vi "ArrangeNodes.vi"() -> ()   [LabVIEW 2016]
uses:
  <resource>/Framework/Providers/Open_GDS/UML/ArrangeNodes/private/localVar.ctl
panel:
  out "Picture":picture
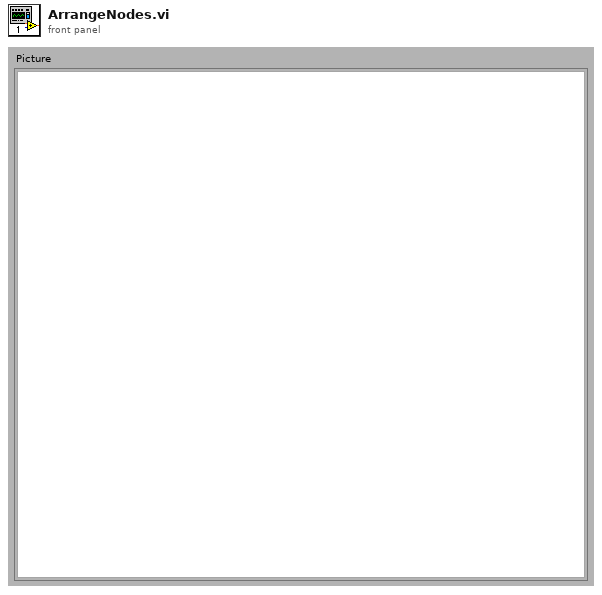
[diagram p1: front panel]
types:
  T1 = typedef "localVar.ctl" = cluster{"nodes":cluster{"x":dbl, "y":dbl, "w":dbl, "h":dbl, "dx":dbl, "dy":dbl, "fixed":bool, "text":string}[], "edges":cluster{"from":i32, "to":i32, "len":dbl}[], "nodeSelected":i32, "bPressed":bool, "NodeRef":u32[]}
  T2 = cluster{"x":dbl, "y":dbl, "w":dbl, "h":dbl, "dx":dbl, "dy":dbl, "fixed":bool, "text":string}[]
  T3 = cluster{"x":dbl, "y":dbl, "w":dbl, "h":dbl, "dx":dbl, "dy":dbl, "fixed":bool, "text":string}
  T4 = cluster{"horizontal":enum16{"left", "center", "right"}, "vertical":enum16{"top", "center", "bottom"}}
  T5 = cluster{"left":i16, "top":i16, "right":i16, "bottom":i16}
  T6 = typedef "LVMouseTypeDef.ctl" = cluster{"Mouse Position":cluster{"X":i32, "Y":i32}, "Mouse Modifiers":cluster{"Button Down":bool, "Shift Mod":bool, "Menu Mod":bool, "Option Mod":bool}}
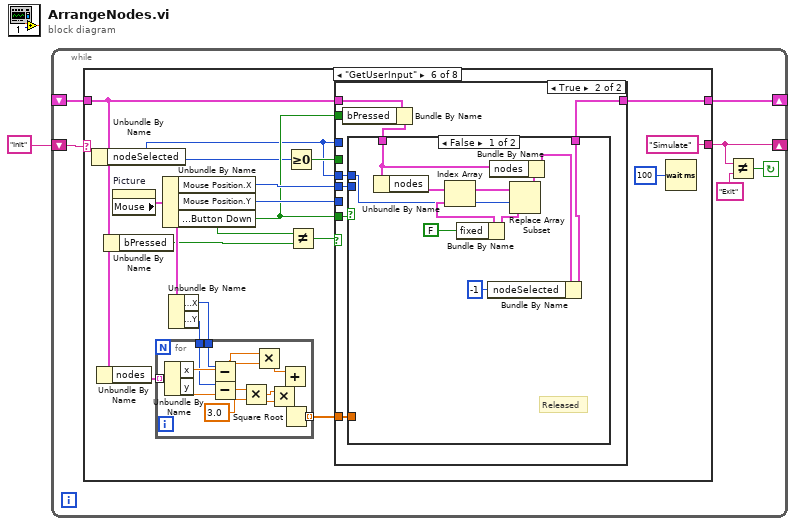
[diagram p0: block diagram]
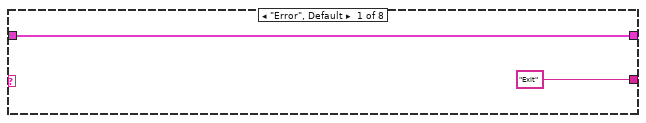
[diagram p2: hidden frame]
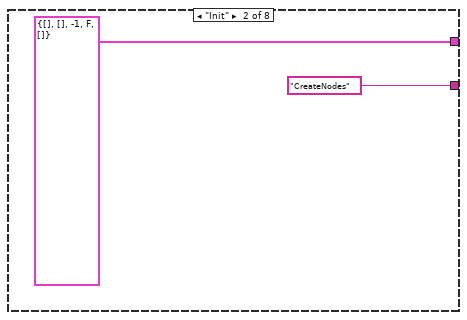
[diagram p3: hidden frame]
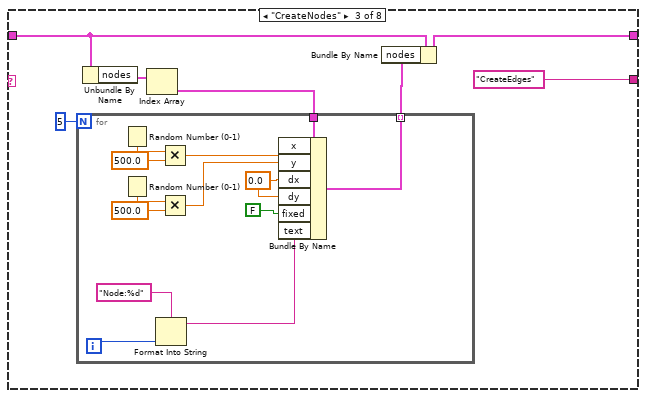
[diagram p4: hidden frame]
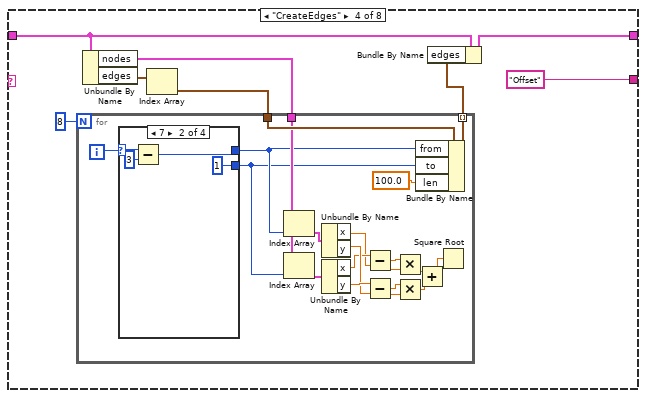
[diagram p5: hidden frame]
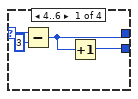
[diagram p6: hidden frame]
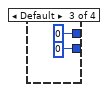
[diagram p7: hidden frame]
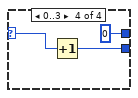
[diagram p8: hidden frame]
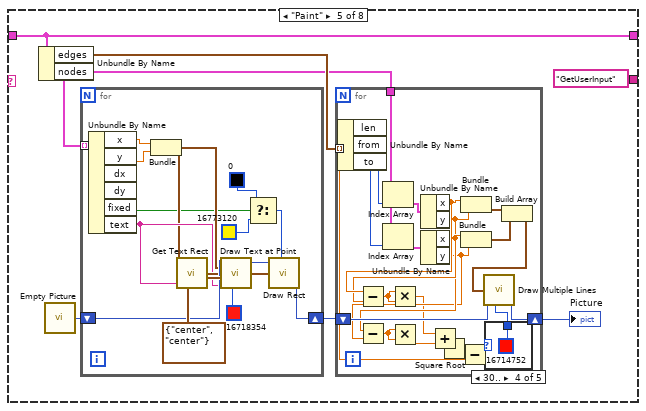
[diagram p9: hidden frame]
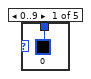
[diagram p10: hidden frame]
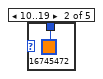
[diagram p11: hidden frame]
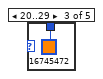
[diagram p12: hidden frame]
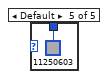
[diagram p13: hidden frame]
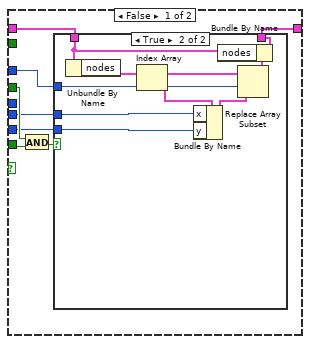
[diagram p14: hidden frame]
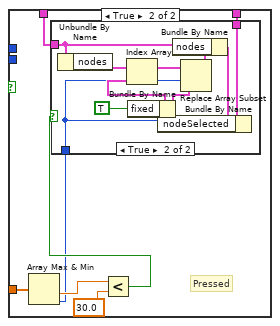
[diagram p16: hidden frame]
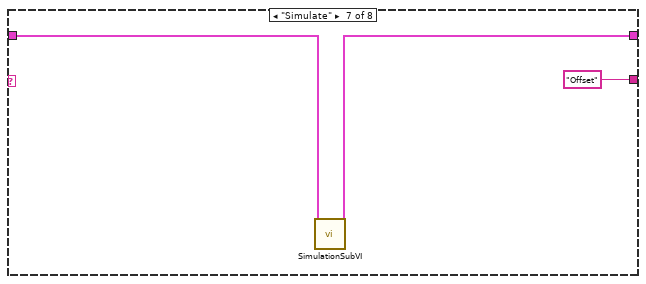
[diagram p18: hidden frame]
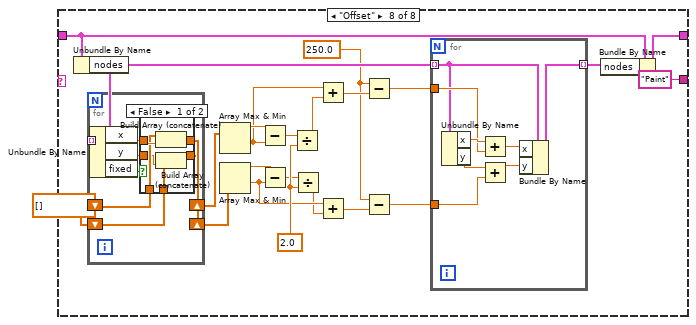
[diagram p19: hidden frame]
diagram:
  n1 = while {
    shift-left: _ -> [w2]
    shift-right: [w3] -> _
    shift-left: "Init" -> [w7]
    shift-right: [w5] -> _
    stop <- w6 continue-if-true
    n2 = case shown="\"GetUserInput\"" w7 {
      tunnel: ["Exit" "CreateNodes" "CreateEdges" "Offset" "GetUserInput" "Simulate" "Offset" "Paint"] -> w5
      tunnel: [w8 T1 {"nodes"=[], "edges"=[], "nodeSelected"=-1, "bPressed"=FALSE, "NodeRef"=[]} ("Cluster") w14 w35 w71 w133 w205 w211] -> w3
      tunnel: w2 -> [w8 _ w15 w36 w71 w131 w206 w212]
      frame "Error", Default {
      }
      frame "Init" {
      }
      frame "CreateNodes" {
        n3 = Unbundle By Name(w15) -> ("nodes"=w17:T2)
        n4 = Index Array(array=w17) -> (element=w16:T3)  [unwired: 1 in]
        n5 = for {
          N: 5 -> [_]
          tunnel: w16 -> [w31]
          tunnel: [w19] -> w13 mode=indexing
          i -> [w28]
          w29 = 0.0 ("dx")
          n6 = Random Number (0-1)() -> (number: 0 to 1=w25:dbl)
          n7 = Random Number (0-1)() -> (number: 0 to 1=w22:dbl)
          n8 = Format Into String(format string="Node:%d" ("Format String"), w28) -> (resulting string=w26:string)  [unwired: 2 in, 1 out]
          n9 = Multiply(x=w25, y=500.0) -> (x*y=w21:dbl)
          n10 = Multiply(x=w22, y=500.0) -> (x*y=w20:dbl)
          n11 = Bundle By Name(cluster=w31, "x"=w21, "y"=w20, "dx"=w29, "dy"=w29, "fixed"=FALSE, "text"=w26) -> (w19:T3)
        }
        n12 = Bundle By Name(cluster=w15, "nodes"=w13) -> (w14:T1)
      }
      frame "CreateEdges" {
        n13 = Unbundle By Name(w36) -> ("nodes"=w32:T2, "edges"=w38:cluster{"from":i32, "to":i32, "len":dbl}[])
        n14 = Index Array(array=w38) -> (element=w37:cluster{"from":i32, "to":i32, "len":dbl})  [unwired: 1 in]
        n15 = for {
          N: 8 -> [_]
          tunnel: w37 -> [w57]
          tunnel: [w56] -> w34 mode=indexing
          tunnel: w32 -> [w55]
          i -> [w43]
          n16 = case shown="7" w43 {
            selector: w43 -> [w61 w65 _ w69]
            tunnel: [w59 w62 0 0] -> w42
            tunnel: [w58 1 0 w68] -> w41
            frame 4..6 {
              n17 = Subtract(x=w61, y=3) -> (x-y=w59:i32)
              n18 = Increment(x=w59) -> (x+1=w58:i32)
            }
            frame 7 {
              n19 = Subtract(x=w65, y=3) -> (x-y=w62:i32)
            }
            frame Default {
            }
            frame 0..3 {
              n20 = Increment(x=w69) -> (x+1=w68:i32)
            }
          }
          n21 = Index Array(array=w55, index=w42) -> (element=w54:T3)
          n22 = Index Array(array=w55, index=w41) -> (element=w53:T3)
          n23 = Unbundle By Name(w54) -> ("x"=w49:dbl, "y"=w51:dbl)
          n24 = Unbundle By Name(w53) -> ("x"=w50:dbl, "y"=w52:dbl)
          n25 = Subtract(x=w50, y=w49) -> (x-y=w48:dbl)
          n26 = Subtract(x=w52, y=w51) -> (x-y=w47:dbl)
          n27 = Multiply(x=w48, y=w48) -> (x*y=w45:dbl)
          n28 = Multiply(x=w47, y=w47) -> (x*y=w46:dbl)
          n29 = Bundle By Name(cluster=w57, "from"=w42, "to"=w41, "len"=100.0) -> (w56:cluster{"from":i32, "to":i32, "len":dbl})
          n30 = Add(x=w45, y=w46) -> (x+y=w44:dbl)
          n31 = Square Root(x=w44) -> ()  [unwired: 1 out]
        }
        n32 = Bundle By Name(cluster=w36, "edges"=w34) -> (w35:T1)
      }
      frame "Paint" {
        n33 = Unbundle By Name(w71) -> ("edges"=w75:cluster{"from":i32, "to":i32, "len":dbl}[], "nodes"=w74:T2)
        n34 = call "Empty Picture"() -> ("empty picture"=w77:picture)
        n35 = for {
          tunnel: w74 -> [w121] mode=indexing
          shift-right: [w115] -> w76
          shift-left: w77 -> [w117]
          w118 = T4 {"horizontal"=enum."center", "vertical"=enum."center"} ("alignment(left, top)")
          n36 = Unbundle By Name(w121) -> ("x"=w120:dbl, "y"=w119:dbl, "fixed"=w110:bool, "text"=w112:string)  [unwired: 2 out]
          n37 = Bundle("x"=w120, "y"=w119) -> (w111:cluster{"x":dbl, "y":dbl})  [unwired: 1 out]
          n38 = call <vilib>:"Get Text Rect.vi"("alignment(left, top)"=w118, "origin(0,0)"=w111, "text"=w112) -> ("rect"=w114:T5)  [unwired: 3 in, 3 out]
          n39 = call <vilib>:"Draw Text at Point.vi"("text color(black)"=u32 16718354, "text"=w112, "alignment(left, top)"=w118, "origin"=w111, "picture"=w117) -> ("new picture"=w116:picture)  [unwired: 4 in, 2 out]
          n40 = Select(t=u32 0, s=w110, f=u32 16773120) -> (s? t:f=w107:u32)
          n41 = call <vilib>:"Draw Rect.vi"("picture"=w116, "rect"=w114, "color(black)"=w107) -> ("new picture"=w115:picture)  [unwired: 2 in, 4 out]
        }
        n42 = for {
          shift-right: [w90] -> w73
          shift-left: w76 -> [w91]
          tunnel: w75 -> [w101] mode=indexing
          tunnel: w74 -> [w100]
          n43 = Unbundle By Name(w101) -> ("len"=w78:dbl, "from"=w97:i32, "to"=w96:i32)
          n44 = Index Array(array=w100, index=w97) -> (element=w99:T3)
          n45 = Index Array(array=w100, index=w96) -> (element=w98:T3)
          n46 = Unbundle By Name(w99) -> ("x"=w89:dbl, "y"=w87:dbl)
          n47 = Unbundle By Name(w98) -> ("x"=w88:dbl, "y"=w86:dbl)
          n48 = Subtract(x=w89, y=w88) -> (x-y=w85:dbl)
          n49 = Subtract(x=w87, y=w86) -> (x-y=w84:dbl)
          n50 = Multiply(x=w85, y=w85) -> (x*y=w82:dbl)
          n51 = Multiply(x=w84, y=w84) -> (x*y=w83:dbl)
          n52 = Add(x=w82, y=w83) -> (x+y=w81:dbl)
          n53 = Square Root(x=w81) -> (sqrt(x)=w79:dbl)
          n54 = Subtract(x=w79, y=w78) -> (x-y=w80:dbl)
          n55 = Bundle("x"=w89, "y"=w87) -> (w95:cluster{"x":dbl, "y":dbl})  [unwired: 1 out]
          n56 = Bundle("x"=w88, "y"=w86) -> (w94:cluster{"x":dbl, "y":dbl})  [unwired: 1 out]
          n57 = case shown="30.." w80 {
            tunnel: [u32 0 u32 16745472 u32 16745472 u32 16714752 u32 11250603] -> w92
            frame 0..9 {
            }
            frame 10..19 {
            }
            frame 20..29 {
            }
            frame 30.. {
            }
            frame Default {
            }
          }
          n58 = Build Array(w95, w94) -> (w93:cluster{"x":dbl, "y":dbl}[])
          n59 = call <vilib>:"Draw Multiple Lines.vi"("picture"=w91, "line endpoints"=w93, "color(black)"=w92) -> ("new picture"=w90:picture)  [unwired: 2 in, 4 out]
        }
        "Picture" <- w73
      }
      frame "GetUserInput" {
        n60 = Unbundle By Name(w131) -> ("nodeSelected"=w126:i32)
        n61 = Unbundle By Name(w131) -> ("nodes"=w124:T2)
        n62 = Unbundle By Name(w131) -> ("bPressed"=w132:bool)
        n63 = property on="Picture" class="Pict"() -> ("Mouse"=w135:T6)  [unwired: 2 in, 2 out]
        n64 = Unbundle By Name(w135) -> ("Mouse Position.X"=w129:i32, "Mouse Position.Y"=w128:i32, "Mouse Modifiers.Button Down"=w127:bool)
        n65 = Unbundle By Name(w135) -> ("Mouse Position.X"=w125:i32, "Mouse Position.Y"=w123:i32)
        n66 = for {
          tunnel: w124 -> [w150] mode=indexing
          tunnel: w125 -> [w149]
          tunnel: w123 -> [w147]
          tunnel: [w138] -> w122 mode=indexing
          n67 = Unbundle By Name(w150) -> ("x"=w148:dbl, "y"=w146:dbl)
          n68 = Subtract(x=w149, y=w148) -> (x-y=w143:dbl)
          n69 = Subtract(x=w147, y=w146) -> (x-y=w145:dbl)
          n70 = Multiply(x=w145, y=3.0) -> (x*y=w142:dbl)
          n71 = Multiply(x=w143, y=w143) -> (x*y=w140:dbl)
          n72 = Multiply(x=w142, y=w142) -> (x*y=w141:dbl)
          n73 = Add(x=w140, y=w141) -> (x+y=w139:dbl)
          n74 = Square Root(x=w139) -> (sqrt(x)=w138:dbl)
        }
        n75 = Greater Or Equal To 0?(x=w126) -> (x >= 0?=w130:bool)
        n76 = Not Equal?(x=w127, y=w132) -> (x != y?=w134:bool)
        n77 = case shown="True" w134 {
          tunnel: w131 -> [w152 w175]
          tunnel: [w151 w172] -> w133
          tunnel: w127 -> [w158 w176]
          tunnel: w130 -> [w157 _]
          tunnel: w129 -> [w155 w170]
          tunnel: w128 -> [w154 _]
          tunnel: w126 -> [w153 _]
          tunnel: w127 -> [_ w174]
          tunnel: w126 -> [_ w171]
          tunnel: w122 -> [_ w169]
          frame False {
            n78 = And(x=w157, y=w158) -> (x .and. y?=w156:bool)
            n79 = case shown="True" w156 {
              tunnel: w152 -> [w159 w162]
              tunnel: w155 -> [_ w167]
              tunnel: w154 -> [_ w166]
              tunnel: w153 -> [_ w163]
              tunnel: [w159 w160] -> w151
              frame False {
              }
              frame True {
                n80 = Unbundle By Name(w162) -> ("nodes"=w168:T2)
                n81 = Index Array(array=w168, index=w163) -> (element=w164:T3)
                n82 = Bundle By Name(cluster=w164, "x"=w167, "y"=w166) -> (w165:T3)
                n83 = Replace Array Subset(array=w168, new element=w165, index=w163) -> (w161:T2)
                n84 = Bundle By Name(cluster=w162, "nodes"=w161) -> (w160:T1)
              }
            }
          }
          frame True {
            n85 = Bundle By Name(cluster=w175, "bPressed"=w174) -> (w173:T1)
            n86 = case shown="False" w176 {
              tunnel: w173 -> [w181 w193]
              tunnel: [w178 w192] -> w172
              tunnel: w171 -> [w180 _]
              tunnel: w170 -> [_ _]
              tunnel: w169 -> [_ w191]
              frame False {
                # "Released"
                n87 = Unbundle By Name(w181) -> ("nodes"=w186:T2)
                n88 = Index Array(array=w186, index=w180) -> (element=w183:T3)
                n89 = Bundle By Name(cluster=w183, "fixed"=FALSE) -> (w184:T3)
                n90 = Replace Array Subset(array=w186, new element=w184, index=w180) -> (w182:T2)
                n91 = Bundle By Name(cluster=w181, "nodes"=w182) -> (w179:T1)
                n92 = Bundle By Name(cluster=w179, "nodeSelected"=-1) -> (w178:T1)
              }
              frame True {
                # "Pressed"
                n93 = Array Max & Min(array=w191) -> (min value=w190:dbl, min index (indices)=w187:i32)  [unwired: 2 out]
                n94 = Less?(x=w190, y=30.0) -> (x < y?=w188:bool)
                n95 = case shown="True" w188 {
                  tunnel: w193 -> [w194 w198]
                  tunnel: [w194 w196] -> w192
                  tunnel: w187 -> [_ w195]
                  frame False {
                  }
                  frame True {
                    n96 = Unbundle By Name(w198) -> ("nodes"=w203:T2)
                    n97 = Index Array(array=w203, index=w195) -> (element=w200:T3)
                    n98 = Bundle By Name(cluster=w200, "fixed"=TRUE) -> (w201:T3)
                    n99 = Replace Array Subset(array=w203, new element=w201, index=w195) -> (w199:T2)
                    n100 = Bundle By Name(cluster=w198, "nodes"=w199) -> (w197:T1)
                    n101 = Bundle By Name(cluster=w197, "nodeSelected"=w195) -> (w196:T1)
                  }
                }
              }
            }
          }
        }
        n102 = Wait (ms)(milliseconds to wait=u32 100) -> ()  [unwired: 1 out]
      }
      frame "Simulate" {
        n103 = call <resource>:"SimulationSubVI.vi"("varIn"=w206) -> ("varOut"=w205:T1)  [unwired: 18 out]
      }
      frame "Offset" {
        w208 = dbl[] []
        w216 = 250.0 ("y")
        w222 = 2.0 ("y")
        n104 = Unbundle By Name(w212) -> ("nodes"=w227:T2)
        n105 = for {
          tunnel: w227 -> [w244] mode=indexing
          shift-right: [w238] -> w209
          shift-left: w208 -> [w240]
          shift-right: [w237] -> w207
          shift-left: w208 -> [w239]
          n106 = Unbundle By Name(w244) -> ("x"=w242:dbl, "y"=w241:dbl, "fixed"=w243:bool)
          n107 = case shown="False" w243 {
            tunnel: w242 -> [w250 _]
            tunnel: w241 -> [w247 _]
            tunnel: [w248 w252] -> w238
            tunnel: [w245 w251] -> w237
            tunnel: w240 -> [w249 w252]
            tunnel: w239 -> [w246 w251]
            frame False {
              n108 = Build Array (concatenate)(w249, w250) -> (w248:dbl[])
              n109 = Build Array (concatenate)(w246, w247) -> (w245:dbl[])
            }
            frame True {
            }
          }
        }
        n110 = Array Max & Min(array=w209) -> (max value=w226:dbl, min value=w224:dbl)  [unwired: 2 out]
        n111 = Array Max & Min(array=w207) -> (max value=w225:dbl, min value=w219:dbl)  [unwired: 2 out]
        n112 = Subtract(x=w226, y=w224) -> (x-y=w223:dbl)
        n113 = Subtract(x=w225, y=w219) -> (x-y=w221:dbl)
        n114 = Divide(x=w223, y=w222) -> (x/y=w220:dbl)
        n115 = Divide(x=w221, y=w222) -> (x/y=w218:dbl)
        n116 = Add(x=w224, y=w220) -> (x+y=w217:dbl)
        n117 = Add(x=w219, y=w218) -> (x+y=w215:dbl)
        n118 = Subtract(x=w216, y=w217) -> (x-y=w214:dbl)
        n119 = Subtract(x=w216, y=w215) -> (x-y=w213:dbl)
        n120 = for {
          tunnel: w227 -> [w232] mode=indexing
          tunnel: w214 -> [w235]
          tunnel: w213 -> [w233]
          tunnel: [w229] -> w210 mode=indexing
          n121 = Unbundle By Name(w232) -> ("x"=w236:dbl, "y"=w234:dbl)
          n122 = Add(x=w236, y=w235) -> (x+y=w231:dbl)
          n123 = Add(x=w234, y=w233) -> (x+y=w230:dbl)
          n124 = Bundle By Name(cluster=w232, "x"=w231, "y"=w230) -> (w229:T3)
        }
        n125 = Bundle By Name(cluster=w212, "nodes"=w210) -> (w211:T1)
      }
    }
    n126 = Not Equal?(x=w5, y="Exit") -> (x != y?=w6:bool)
  }
